vi "Read tipo_generador.vi"(8 "error in (no error)":errorcluster, 11 "Prueba01 in":refnum<class "Prueba01.lvclass">) -> (0 "error out":errorcluster, 2 "tipo_generador":string, 3 "Prueba01 out":refnum<class "Prueba01.lvclass">)   [LabVIEW 2019, in "Prueba01.lvclass"]
uses:
  Prueba01.lvclass
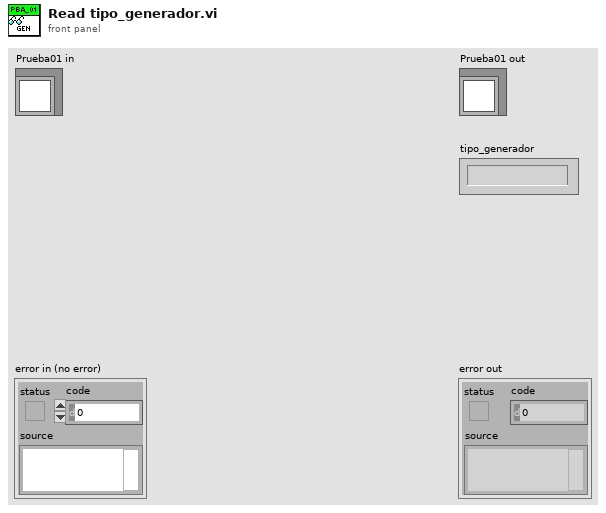
[diagram p1: front panel]
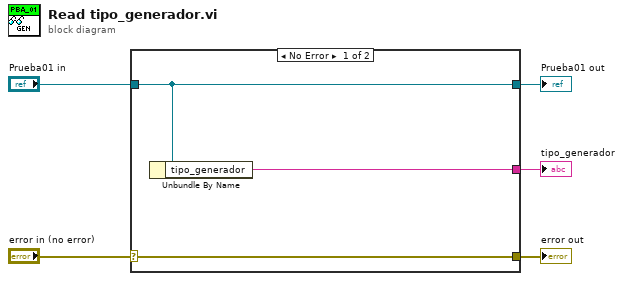
[diagram p0: block diagram]
diagram:
  n1 = case shown="No Error" "error in (no error)" {
    selector: "error in (no error)" -> [w8 w9]
    tunnel: [w8 w9] -> w4
    tunnel: [w7 w10] -> w2
    tunnel: "Prueba01 in" -> [w7 w10]
    tunnel: [w6 _] -> w1
    frame No Error {
      n2 = Unbundle By Name(w7) -> ("tipo_generador"=w6:string)
    }
    frame Error {
    }
  }
  "error out" <- w4
  "Prueba01 out" <- w2
  "tipo_generador" <- w1
